vi "QueryDepartments.vi"(8 "error in (no error)":errorcluster, 10 "TableName(\"\")":string, 11 "ExcuseNotes in":refnum<class "ExcuseNotesHandler.lvclass">) -> (0 "error out":errorcluster, 2 "Departments(\"\")":string[](array[string]), 3 "ExcuseNotes out":refnum<class "ExcuseNotesHandler.lvclass">)   [LabVIEW 2015, in "ExcuseNotesHandler.lvclass"]
uses:
  ExcuseNotesHandler.lvclass
  ExcuseNotesHandler.lvclass/ExcuseNotesHandler.ctl
  API/_Database/Database.lvclass
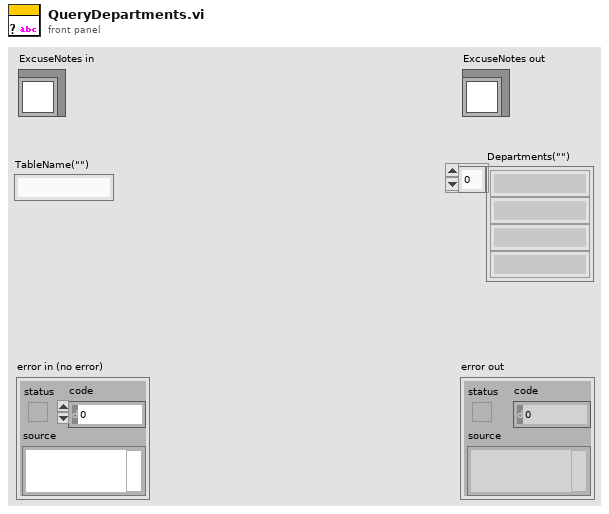
[diagram p1: front panel]
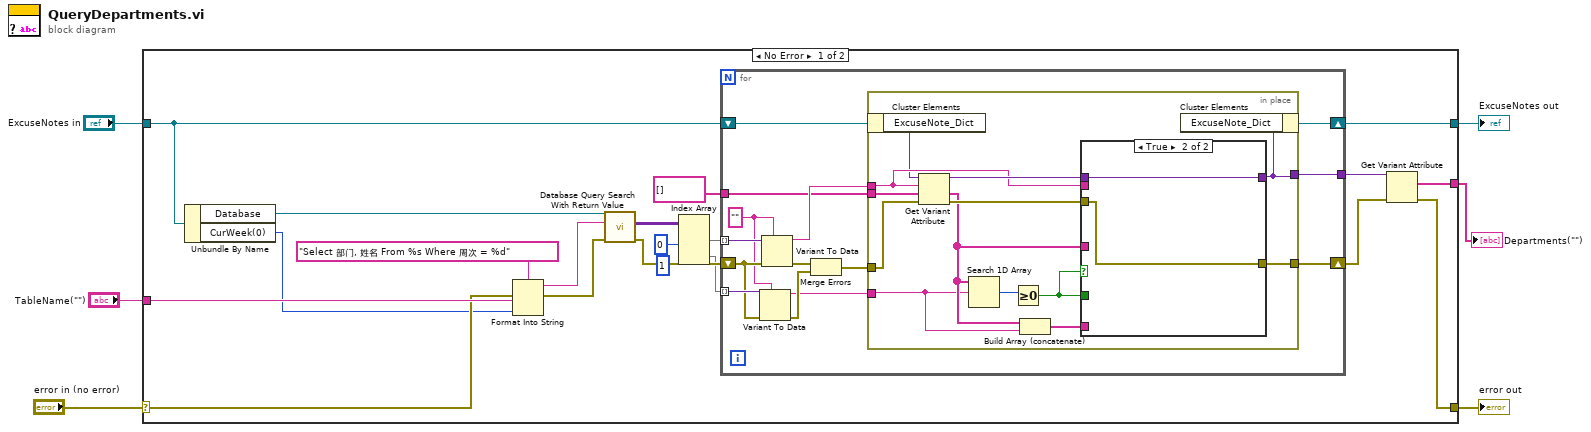
[diagram p0: block diagram]
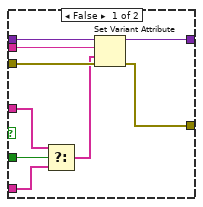
[diagram p2: hidden frame]
diagram:
  n1 = case shown="No Error" "error in (no error)" {
    selector: "error in (no error)" -> [w22 w66]
    tunnel: [w8 w66] -> w5
    tunnel: [w11 w65] -> w3
    tunnel: "ExcuseNotes in" -> [w15 w65]
    tunnel: "TableName(\"\")" -> [w23 _]
    tunnel: [w7 _] -> w1
    frame No Error {
      n2 = Unbundle By Name(w15) -> ("Database"=w26:refnum<class "Database.lvclass">, "CurWeek(0)"=w16:i32)
      n3 = Format Into String(format string="Select 部门, 姓名 From %s Where 周次 = %d" ("SQL query"), error in=w22, w23, w16) -> (resulting string=w24:string, error out=w21:errorcluster)  [unwired: 1 in]
      n4 = call "Database Query Search With Return Value.vi"("error in (no error)"=w21, "SQL query"=w24, "object in"=w26) -> ("error out"=w17:errorcluster, "recordset data"=w20:variant[][])  [unwired: 5 in, 2 out]
      n5 = Index Array(array=w20, index (col) #1=0 ("disabled index (col)"), index (col) #2=1 ("index (col)")) -> (element #1=w18:variant[], element #2=w13:variant[])  [unwired: 2 in]
      n6 = for {
        tunnel: w18 -> [w40] mode=indexing
        shift-right: [w28] -> w9
        shift-left: w17 -> [w37]
        tunnel: w13 -> [w38] mode=indexing
        tunnel: string[] [] -> [w32]
        shift-right: [w29] -> w11
        shift-left: w15 -> [w39]
        tunnel: [w27] -> w10
        w36 = ""
        n7 = Variant To Data(error in=w37, type=w36, Variant=w38) -> (data=w30:string, error out=w34:errorcluster)
        n8 = Variant To Data(error in=w37, type=w36, Variant=w40) -> (data=w33:string, error out=w35:errorcluster)
        n9 = Merge Errors(w35, w34) -> (w31:errorcluster)
        n10 = in-place {
          in-place-border: w33 -> [w49]
          in-place-border: w32 -> [w53]
          in-place-border: w31 -> [w52]
          in-place-border: w30 -> [w45]
          in-place-border: [w48] -> w28
          in-place-border: [w43] -> w27
          n11 = in-place-cluster #1(w39) -> ("ExcuseNote_Dict"=w42:variant)
          n12 = Get Variant Attribute(Variant=w42, name=w49, default value (empty Variant)=w53, error in=w52) -> (duplicate Variant=w51:variant, value=w46:string[], error out=w50:errorcluster)  [unwired: 1 out]
          n13 = Search 1D Array(1D array=w46, element=w45) -> (index of element=w47:i32)  [unwired: 1 in]
          n14 = Greater Or Equal To 0?(x=w47) -> (x >= 0?=w41:bool)
          n15 = Build Array (concatenate)(w46, w45) -> (w44:string[])
          n16 = case shown="True" w41 {
            tunnel: w51 -> [w62 w64]
            tunnel: w50 -> [w61 w63]
            tunnel: w49 -> [w60 _]
            tunnel: [w59 w63] -> w48
            tunnel: w41 -> [w58 _]
            tunnel: w46 -> [w57 _]
            tunnel: w44 -> [w56 _]
            tunnel: [w54 w64] -> w43
            frame False {
              n17 = Select(t=w57, s=w58, f=w56) -> (s? t:f=w55:string[])
              n18 = Set Variant Attribute(Variant=w62, name=w60, value=w55, error in=w61) -> (Variant out=w54:variant, error out=w59:errorcluster)  [unwired: 1 out]
            }
            frame True {
            }
          }
          n19 = in-place-cluster #1("ExcuseNote_Dict"=w43) -> (w29:refnum<class "ExcuseNotesHandler.lvclass">)
        }
      }
      n20 = Get Variant Attribute(Variant=w10, error in=w9) -> (names=w7:string[], error out=w8:errorcluster)  [unwired: 2 in, 2 out]
    }
    frame Error {
    }
  }
  "error out" <- w5
  "ExcuseNotes out" <- w3
  "Departments(\"\")" <- w1
